vi "MCSMain.vi"(5 "nOfBins":u32) -> (14 "abortOrTimeOut":bool)   [LabVIEW 2014]
uses:
  <vilib>/Platform/TimedLoop/XDataNode/timing_clust.ctl
  <vilib>/Platform/TimedLoop/XDataNode/nitl_modes.ctl
  <vilib>/Platform/TimedLoop/XDataNode/wakeup.ctl
  Controls/infoHandle.ctl
  <vilib>/rvi/Emulation/niFpgaSctlEmulationGetInTimedLoop.vi
  <vilib>/rvi/Emulation/niFpgaEmulationReportErrorSimple.vi
  <vilib>/rvi/Emulation/niFpgaGetClockAttributes.vi
  <vilib>/rvi/Emulation/niFpgaCriticalErrorInLSC.vi
  Sequencer/sequencerGlobVars.vi
  <vilib>/rvi/eio/common/nirviEmuTemplateMethod_errors.vi
  <vilib>/Platform/TimedLoop/XDataNode/XDataNode.xnode
  <vilib>/eio/EIONode/EIONode.xnode
  <vilib>/Platform/TimedLoop/XDataNode/XDNodeRunTimeDep.lvlib
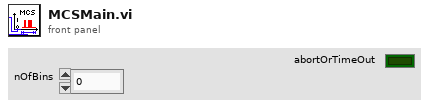
[diagram p1: front panel]
types:
  T1 = typedef "XDNodeRunTimeDep.lvlib/timing_clust.ctl" = cluster{"Expected End [f-1]":u64, "Actual End [f-1]":u64, "Finished Late? [f-1]":bool, "Expected End [i-1]":u64, "Actual End [i-1]":u64, "Finished Late? [i-1]":bool, "Expected Start [i]":u64, "Actual Start [i]":u64, "Expected Start [f]":u64, "Actual Start [f]":u64, "Source Name":string, "Structure Name":string, "Period":i64, "Deadline":i64, "Offset":i64, "Start":i64, "Priority":i32, "Timeout":i32, "Mode":T2, "Wakeup Reason":T3, "Error":errorcluster, "Source Type":string, "Secondary Source Type":string, "Global End Time":u64, "Global Start Time":u64, "Frame Duration":u64, "Iteration Duration":u64, "Assigned CPU":i32, "I/O Scan Engine Mode":u32}
  T2 = typedef "XDNodeRunTimeDep.lvlib/nitl_modes.ctl" = enum32{"No Change", "Process missed periods, maintain original phase", "Discard missed periods, maintain original phase", "Process missed periods, ignore original phase", "Discard missed periods, ignore original phase"}
  T3 = typedef "XDNodeRunTimeDep.lvlib/wakeup.ctl" = enum32{"Normal", "Aborted", "Asynchronous wakeup", "Timing source error", "Timed loop error", "Timeout"}
  T4 = typedef "infoHandle.ctl" = enum16{"abortedScan", "stepComplete", "newScan", "newBunch", "preparingStep"}
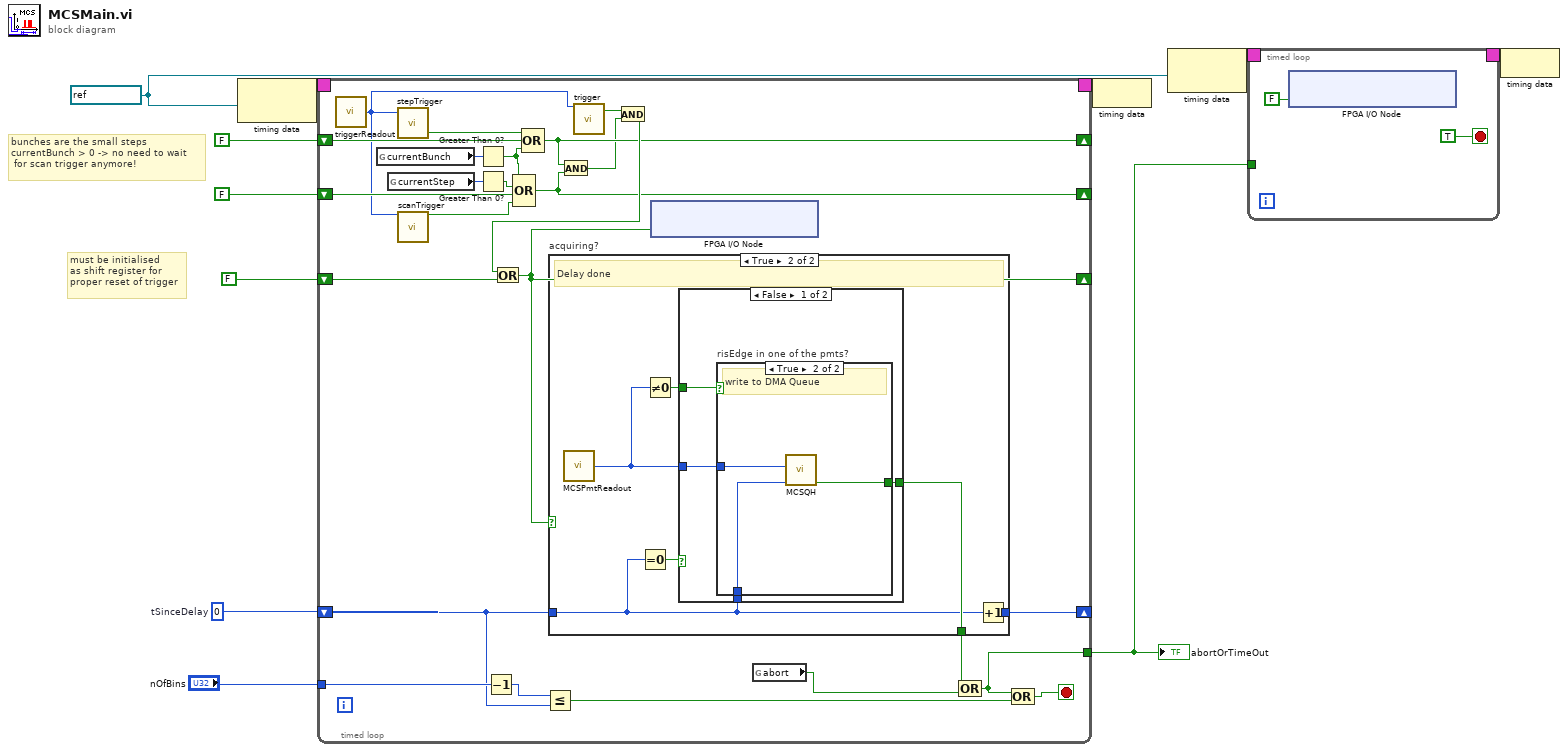
[diagram p0: block diagram]
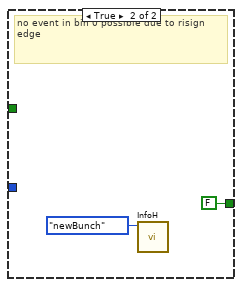
[diagram p4: hidden frame]
diagram:
  w9 = u32 0  # tSinceDelay
  w5 = refnum<k21> "100MHz" ("Source Name")
  # "bunches are the small steps\ncurrentBunch > 0 -> no need to wait\n for scan trigger anymore!"
  # "must be initialised\nas shift register for\nproper reset of trigger"
  n1 = node-c288(w5) -> (w11:T1)
  n2 = timed-loop {
    timing: w11 -> [_]
    timing-out: [_] -> w10
    shift-right: [w36] -> _
    shift-left: w9 -> [w33]
    tunnel: "nOfBins" -> [w35]
    tunnel: [w28] -> w4
    shift-right: [w24] -> _
    shift-left: FALSE ("triggered") -> [w27]
    shift-right: [w14] -> _
    shift-left: FALSE -> [w22]
    shift-right: [w15] -> _
    shift-left: FALSE -> [w20]
    stop <- w30 stop-if-true
    n3 = call "triggerReadout.vi"() -> ("triggerReadout"=w17:u16)
    n4 = global read "sequencerGlobVars.vi" "currentBunch"() -> (w21:i32)
    n5 = global read "sequencerGlobVars.vi" "currentStep"() -> (w26:i32)
    n6 = call "stepTrigger.vi"("triggerReadout"=w17) -> ("triggeredScan"=w16:bool)  [unwired: 18 in]
    n7 = call "scanTrigger.vi"("triggerReadout"=w17) -> ("triggeredScan"=w23:bool)  [unwired: 18 in]
    n8 = Greater Than 0?(x=w21) -> (x > 0?=w12:bool)
    n9 = Greater Than 0?(x=w26) -> (x > 0?=w25:bool)
    n10 = Decrement(x=w35) -> (x-1=w34:u32)
    n11 = Compound Arithmetic op=OR(w12, w25, w22, w23) -> (w14:bool)
    n12 = Compound Arithmetic op=OR(w16, w20, w12) -> (w15:bool)
    n13 = Less Or Equal?(x=w34, y=w33) -> (x <= y?=w29:bool)
    n14 = And(x=w15, y=w14) -> (x .and. y?=w13:bool)
    n15 = call "trigger.vi"("triggerReadout"=w17) -> ("triggered"=w19:bool)  [unwired: 18 in]
    n16 = And(x=w19, y=w13) -> (x .and. y?=w18:bool)
    n17 = Or(x=w18, y=w27) -> (x .or. y?=w24:bool)
    n18 = case "acquiring?" shown="True" w24 {
      tunnel: w33 -> [w37 w38]
      tunnel: [w37 w43] -> w36
      tunnel: [_ w40] -> w32
      frame False {
      }
      frame True {
        # "Delay done"
        n19 = call "MCSPmtReadout.vi"() -> ("pmtOut"=w41:u8)  [unwired: 5 in]
        n20 = Equal To 0?(x=w38) -> (x = 0?=w39:bool)
        n21 = Not Equal To 0?(x=w41) -> (x != 0?=w42:bool)
        n22 = case shown="False" w39 {
          tunnel: w42 -> [w47 _]
          tunnel: w41 -> [w46 _]
          tunnel: w38 -> [w45 _]
          tunnel: [w44 FALSE ("MCSWriteTimeout")] -> w40
          frame False {
            n23 = case "risEdge in one of the pmts?" shown="True" w47 {
              tunnel: w46 -> [_ w49]
              tunnel: w45 -> [_ w50]
              tunnel: [_ w48] -> w44
              frame False {
              }
              frame True {
                # "write to DMA Queue"
                n24 = call "MCSQH.vi"("TimeStamp"=w50, "activePMT"=w49) -> ("MCSWriteTimeout"=w48:bool)  [unwired: 9 in]
              }
            }
          }
          frame True {
            # "no event in bin 0 possible due to risign edge"
            n25 = call "InfoH.vi"("info"=infoHandle."newBunch") -> ()  [unwired: 11 in]
          }
        }
        n26 = Increment(x=w38) -> (x+1=w43:u32)
      }
    }
    n27 = xnode "FPGA I/O Node"("MCSScanFlagDio9Con1"=w24) -> ()  [unwired: 1 in, 1 out]
    n28 = global read "sequencerGlobVars.vi" "abort"() -> (w31:bool)
    n29 = Compound Arithmetic op=OR(w32, w31) -> (w28:bool)
    n30 = Compound Arithmetic op=OR(w28, w29) -> (w30:bool)
  }
  "abortOrTimeOut" <- w4
  n31 = node-c288(w10) -> ()
  n32 = node-c288(w5) -> (w7:T1)
  n33 = timed-loop {
    timing: w7 -> [_]
    timing-out: [_] -> w6
    tunnel: w4 -> [_]
    stop <- TRUE stop-if-true
    n34 = xnode "FPGA I/O Node"("MCSScanFlagDio9Con1"=FALSE) -> ()  [unwired: 1 in, 1 out]
  }
  n35 = node-c288(w6) -> ()
